vi "RichToFlatnixnet_grpc_WriteSignalXYRequest.vi"(5 "OutputClusterType":T1, 11 "InputCluster":T4) -> (3 "OutputCluster":T1)   [LabVIEW 2025, in "xnet-grpc_client.lvlib"]
uses:
  xnet-grpc_client.lvlib
  nixnet_grpc_WriteSignalXYRequest.ctl
  nixnet_grpc_WriteSignalXYRequest_timeout_enum/nixnet_grpc_WriteSignalXYRequest_timeout_enum.lvclass
  nidevice_grpc_Session.ctl
  nixnet_grpc_WriteSignalXYRequest_Flat.ctl
  nidevice_grpc_Session_Flat.ctl
  nixnet_grpc_TimeOut.ctl
  nixnet_grpc_WriteSignalXYRequest_timeout_enum/nixnet_grpc_WriteSignalXYRequest_timeout_enum.lvclass/nixnet_grpc_WriteSignalXYRequest_timeout_enum.ctl
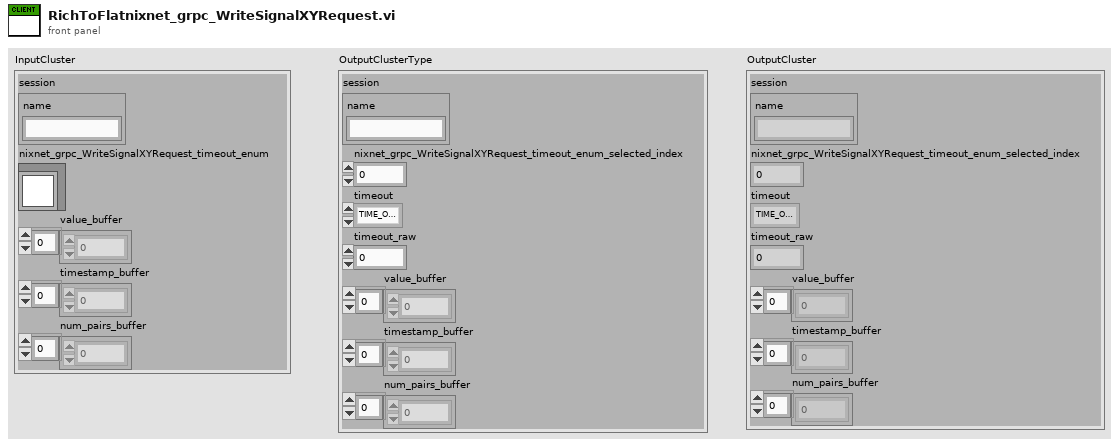
[diagram p1: front panel]
types:
  T1 = typedef "xnet-grpc_client.lvlib/nixnet_grpc_WriteSignalXYRequest_Flat.ctl" = cluster{"session":T2, "nixnet_grpc_WriteSignalXYRequest_timeout_enum_selected_index":i32, "timeout":T3, "timeout_raw":dbl, "value_buffer":dbl[], "timestamp_buffer":u64[], "num_pairs_buffer":u32[]}
  T2 = typedef "xnet-grpc_client.lvlib/nidevice_grpc_Session_Flat.ctl" = cluster{"name":string}
  T3 = typedef "xnet-grpc_client.lvlib/nixnet_grpc_TimeOut.ctl" = enum32{"TIME_OUT_NONE", "TIME_OUT_INFINITE"}
  T4 = typedef "xnet-grpc_client.lvlib/nixnet_grpc_WriteSignalXYRequest.ctl" = cluster{"session":T5, "nixnet_grpc_WriteSignalXYRequest_timeout_enum":refnum<class "nixnet_grpc_WriteSignalXYRequest_timeout_enum.lvclass">, "value_buffer":dbl[], "timestamp_buffer":u64[], "num_pairs_buffer":u32[]}
  T5 = typedef "xnet-grpc_client.lvlib/nidevice_grpc_Session.ctl" = cluster{"name":string}
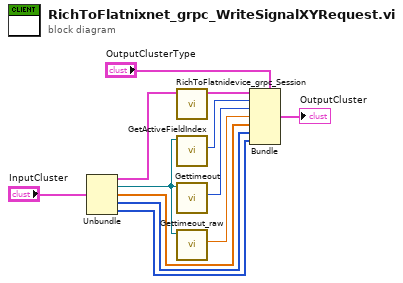
[diagram p0: block diagram]
diagram:
  n1 = Unbundle "Unbundle"("InputCluster") -> ("session"=w9:T5, "nixnet_grpc_WriteSignalXYRequest_timeout_enum"=w7:refnum<class "nixnet_grpc_WriteSignalXYRequest_timeout_enum.lvclass">, "value_buffer"=w3:dbl[], "timestamp_buffer"=w2:u64[], "num_pairs_buffer"=w1:u32[])
  n2 = call "RichToFlatnidevice_grpc_Session.vi"("InputCluster"=w9) -> ("OutputCluster"=w8:T2)  [unwired: 10 in]
  n3 = call "GetActiveFieldIndex.vi"("OneOfTemplate in"=w7) -> ("Active Field Index"=w6:i32)  [unwired: 8 in, 2 out]
  n4 = call "Gettimeout.vi"("OneOfTemplate in"=w7) -> ("Get_Val"=w5:T3)  [unwired: 8 in, 2 out]
  n5 = call "Gettimeout_raw.vi"("OneOfTemplate in"=w7) -> ("Get_Val"=w4:dbl)  [unwired: 8 in, 2 out]
  n6 = Bundle "Bundle"(cluster="OutputClusterType", "session"=w8, "nixnet_grpc_WriteSignalXYRequest_timeout_enum_selected_index"=w6, "timeout"=w5, "timeout_raw"=w4, "value_buffer"=w3, "timestamp_buffer"=w2, "num_pairs_buffer"=w1) -> (→"OutputCluster":T1)
